vi "RP ADC to Volts 1D.vi"(6 "osc_fpga_cnv_cnt_to_v method":bool, 7 "Max Volts":sgl=1.0, 9 "Signal bits":i32=14, 11 "ADC data":i16[](array[numeric])) -> (3 "Volts":sgl[](array[numeric]))   [LabVIEW 2015]
panel:
  out "x << y":i32
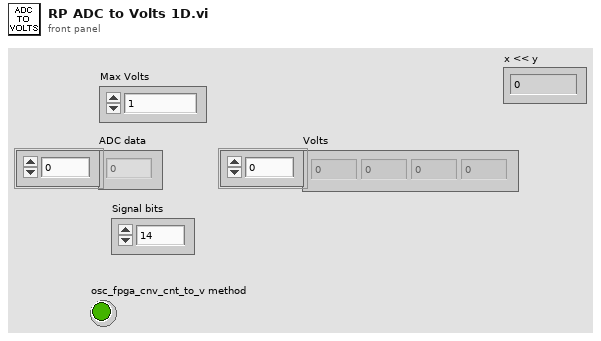
[diagram p1: front panel]
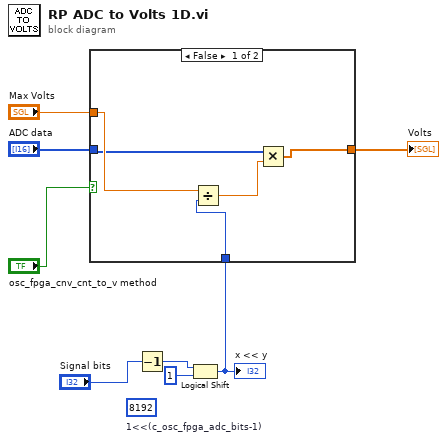
[diagram p0: block diagram]
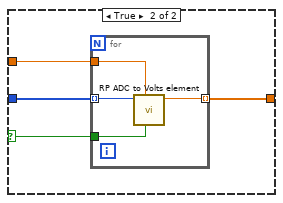
[diagram p2: hidden frame]
diagram:
  (unwired) 8192  # 1<<(c_osc_fpga_adc_bits-1)
  n1 = Decrement(x="Signal bits") -> (x-1=w2:i32)
  n2 = Logical Shift(y=w2, x=1) -> (x << y=w1:i32)
  "x << y" <- w1
  n3 = case shown="False" "osc_fpga_cnv_cnt_to_v method" {
    selector: "osc_fpga_cnv_cnt_to_v method" -> [_ w14]
    tunnel: "ADC data" -> [w11 w17]
    tunnel: [w10 w16] -> w7
    tunnel: "Max Volts" -> [w13 w15]
    tunnel: w1 -> [w9 _]
    frame False {
      n4 = Divide(x=w13, y=w9) -> (x/y=w12:sgl)
      n5 = Multiply(x=w11, y=w12) -> (x*y=w10:sgl[])
    }
    frame True {
      n6 = for {
        tunnel: w17 -> [w21] mode=indexing
        tunnel: [w20] -> w16 mode=indexing
        tunnel: w14 -> [w19]
        tunnel: w15 -> [w18]
        n7 = call "RP ADC to Volts element.vi"("osc_fpga_cnv_cnt_to_v method"=w19, "Max Volts"=w18, "ADC data"=w21) -> ("Volts"=w20:sgl)  [unwired: 8 in]
      }
    }
  }
  "Volts" <- w7
